vi "pixie array size.vi"(8 "error in (no error)":errorcluster, 11 "Pixie input array":u16[](array[numeric])) -> (0 "error out":errorcluster, 1 "Array size":u32[](array[numeric]), 2 "pixie 2d array":u16[][](array[numeric]), 3 "size of pixie array":u32, 5 "number of events":dbl)   [LabVIEW 2016]
doc: "Check pixie array to find the number of non -1 values."
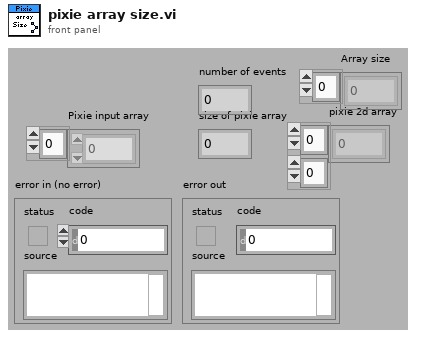
[diagram p1: front panel]
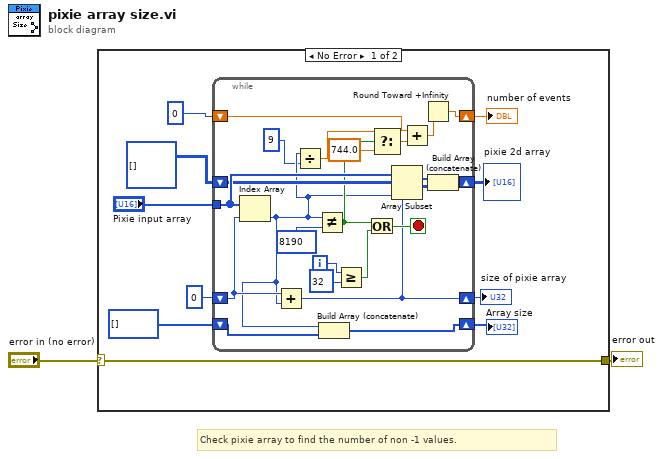
[diagram p0: block diagram]
diagram:
  # "Check pixie array to find the number of non -1 values."
  n1 = case shown="No Error" "error in (no error)" {
    selector: "error in (no error)" -> [w9 w35]
    tunnel: [w9 w35] -> w1
    frame No Error {
      n2 = while {
        tunnel: "Pixie input array" -> [w28]
        shift-right: [w27] -> w10
        shift-left: 0 ("index") -> [w34]
        shift-right: [w25] -> w7
        shift-left: u16[][] [] -> [w24]
        shift-right: [w22] -> w5
        shift-left: u16[] [] -> [w23]
        shift-right: [w13] -> w3
        shift-left: u32 0 ("index") -> [w15]
        i -> [w29]
        stop <- w30 stop-if-true
        n3 = Index Array(array=w28, index=w34) -> (element=w19:u16)
        n4 = Add(x=w34, y=w19) -> (x+y=w27:i32)
        n5 = Divide(x=w19, y=u16 9 ("element")) -> (x/y=w17:dbl)
        n6 = Not Equal?(x=w19, y=u16 8190) -> (x != y?=w21:bool)
        n7 = Build Array (concatenate)(w19, w23) -> (w22:u16[])
        n8 = Greater Or Equal?(x=w29, y=32) -> (x >= y?=w31:bool)
        n9 = Or(x=w21, y=w31) -> (x .or. y?=w30:bool)
        n10 = Select(t=w17, s=w21, f=744.0) -> (s? t:f=w16:dbl)
        n11 = Array Subset(array=w28, index=w27, length=w19) -> (w26:u16[])
        n12 = Add(x=w15, y=w16) -> (x+y=w14:dbl)
        n13 = Round Toward +Infinity(x=w14) -> (ceil(x): smallest int >= x=w13:dbl)
        n14 = Build Array (concatenate)(w26, w24) -> (w25:u16[][])
      }
      "size of pixie array" <- w10
      "pixie 2d array" <- w7
      "Array size" <- w5
      "number of events" <- w3
    }
    frame Error {
    }
  }
  "error out" <- w1
